vi "MatrixVg_Bdep.vi"(0 "B-table String":string, 3 "Time Stamp":timestamp, 6 "Play Button":bool, 7 "Custom Folder":string, 8 "Settings":T2={"Ring 3"=1, "Ring 2"=4, "Fixed Current mkA"=0.5, "If yes, the current is:"=enum."Radio Selection 1", "Ressitance measurements?"=TRUE, "Commute DC current?"=FALSE} {"Ring 3" items=["1 kOhm", "10 kOhm", "100 kOhm", "1 Mohm", "10 mOhm"]; "Ring 2" items=["1 kOhm", "10 kOhm", "100 kOhm", "1 Mohm", "10 MOhm"]}, 9 "Instruments":T3={"Oscillator"=TRUE, "Addr 1 lock-in"=TRUE, "Addr 1 lock-in oop"=TRUE, "Addr 2 lock-in"=TRUE, "Addr 2 lock-in oop"=TRUE, "Addr 3 lock-in"=FALSE, "Addr 3 lock-in oop"=FALSE, "Voltage (Vk1)"=FALSE, "Current (Ik1)"=TRUE, "Voltage (Vk2)"=FALSE, "Current (Ik2)"=FALSE, "Voltage (Vk3)"=FALSE, "Current (Ik3)"=FALSE, "Channel 1 (Vnano1)  "=FALSE, "Channel 2 (Vnano1b)"=FALSE, "Channel 1 (Vnano2)   "=FALSE, "Channel 2 (Vnano2b)"=FALSE, "Thermometer 1 (T1)"=TRUE, "Magnetic Field (B)"=TRUE, "Capacitance (C) and Loss (L)"=FALSE}, 10 "VgCluster":T4={"V1 (V)"=-1.0, "V2 (V)"=1.0, "Sweep rate, V/min"=1.0, "Time btw \npoints, sec"=1.0, "points at each Vg"=1, "Compliance, mkA"=0.05, "No-record rate, V/min"=30.0, "Full sweep?"=FALSE} {"No-record rate, V/min" min=0.0 max=1.0 step=0.01 format="%_4f"; "V2 (V)" min=-4.0 max=4.0 step=0.1 format="%.1f"; "Compliance, mkA" min=0.0 max=1.0 step=0.01 format="%.3f"; "Time btw \npoints, sec" format="%.2f"; "Sweep rate, V/min" min=0.0 max=1.0 step=0.01 format="%_4f"; "V1 (V)" min=-4.0 max=4.0 step=0.1 format="%.1f"}, 11 "BCluster":T1={"Starting B (T)"=-1.0, "Final B (T)"=1.0, "Step (T)"=1.0, "Time for persistant, min"=1.0} {"Final B (T)" min=-4.0 max=4.0 step=0.1 format="%.2f"; "Time for persistant, min" format="%.2f"; "Step (T)" min=0.0 max=1.0 step=0.01 format="%_4f"; "Starting B (T)" min=-4.0 max=4.0 step=0.1 format="%.2f"}) -> ()   [LabVIEW 2017]
uses:
  <vilib>/Utility/file.llb/Read From Spreadsheet File (DBL).vi
panel:
  out "Communication":string
  out "B Array":dbl[](array[numeric])
  out "Experiment ends at:":string
  out "Hours":dbl format="%.1f"
  out "Estimated time of experiment:":i16
  out "ArraySens":i8[](array[numeric])
  out "ArrayOsc":dbl[](array[numeric])
  out "# of configurations":i8
  out "Large Array":bool[][][](array[boolean])
  out "Contact configuration file (*.conf)":path
  # "hours"
  # "min.="
  # "Values of B field can be also entered as the table by copying\nand pasting a column of numbers in a \"B table\" string at the \nfar right side of this window."
  # "Lock-in Amplifiers"
  # "Temperature"
  # "SourceMeters"
  # "Nanovoltmeters"
  # "Main"
  # "(not recommended, too slow)"
  # "Magnetic Field"
  # "Capacitance & Loss"
  # "(not recommended, too slow)"
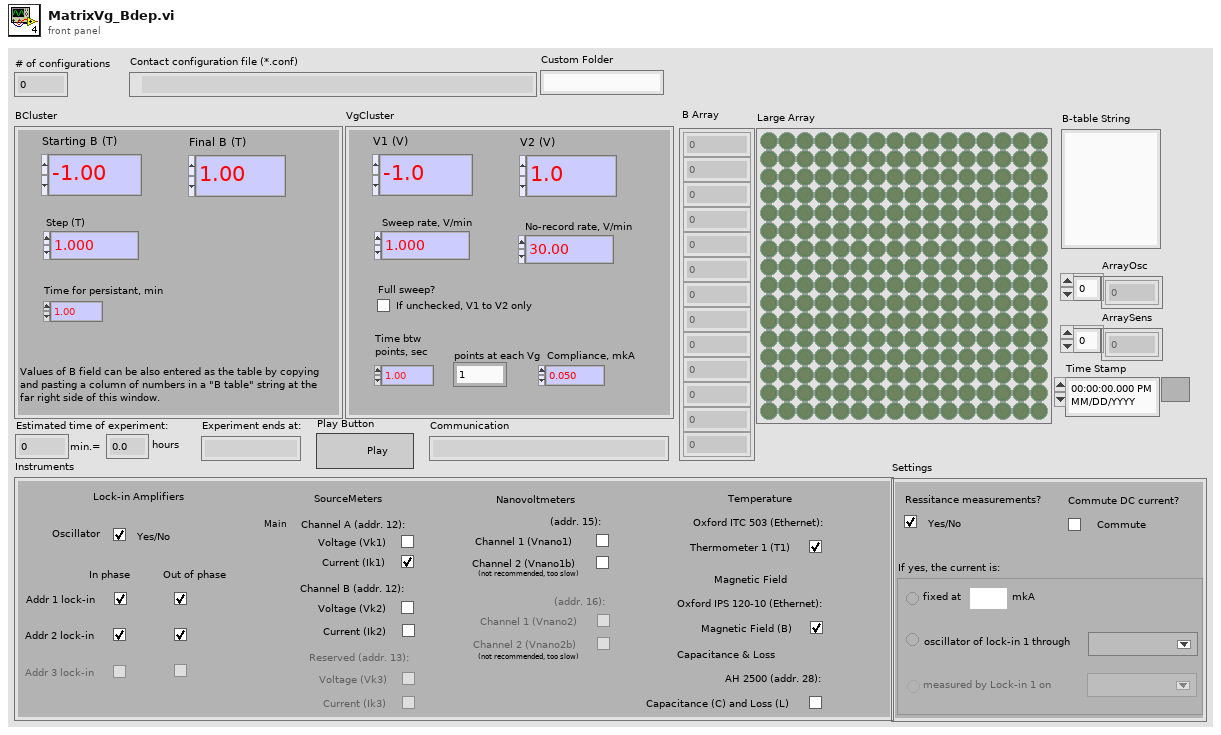
[diagram p1: front panel]
types:
  T1 = cluster{"Starting B (T)":dbl, "Final B (T)":dbl, "Step (T)":dbl, "Time for persistant, min":dbl}
  T2 = cluster{"Ring 3":u16, "Ring 2":u16, "Fixed Current mkA":dbl, "If yes, the current is:":enum32{"Radio Selection 1", "Radio Selection 2", "Radio Selection 3"}, "Ressitance measurements?":bool, "Commute DC current?":bool}
  T3 = cluster{"Oscillator":bool, "Addr 1 lock-in":bool, "Addr 1 lock-in oop":bool, "Addr 2 lock-in":bool, "Addr 2 lock-in oop":bool, "Addr 3 lock-in":bool, "Addr 3 lock-in oop":bool, "Voltage (Vk1)":bool, "Current (Ik1)":bool, "Voltage (Vk2)":bool, "Current (Ik2)":bool, "Voltage (Vk3)":bool, "Current (Ik3)":bool, "Channel 1 (Vnano1)  ":bool, "Channel 2 (Vnano1b)":bool, "Channel 1 (Vnano2)   ":bool, "Channel 2 (Vnano2b)":bool, "Thermometer 1 (T1)":bool, "Magnetic Field (B)":bool, "Capacitance (C) and Loss (L)":bool}
  T4 = cluster{"V1 (V)":dbl, "V2 (V)":dbl, "Sweep rate, V/min":dbl, "Time btw \npoints, sec":dbl, "points at each Vg":i32, "Compliance, mkA":dbl, "No-record rate, V/min":dbl, "Full sweep?":bool}
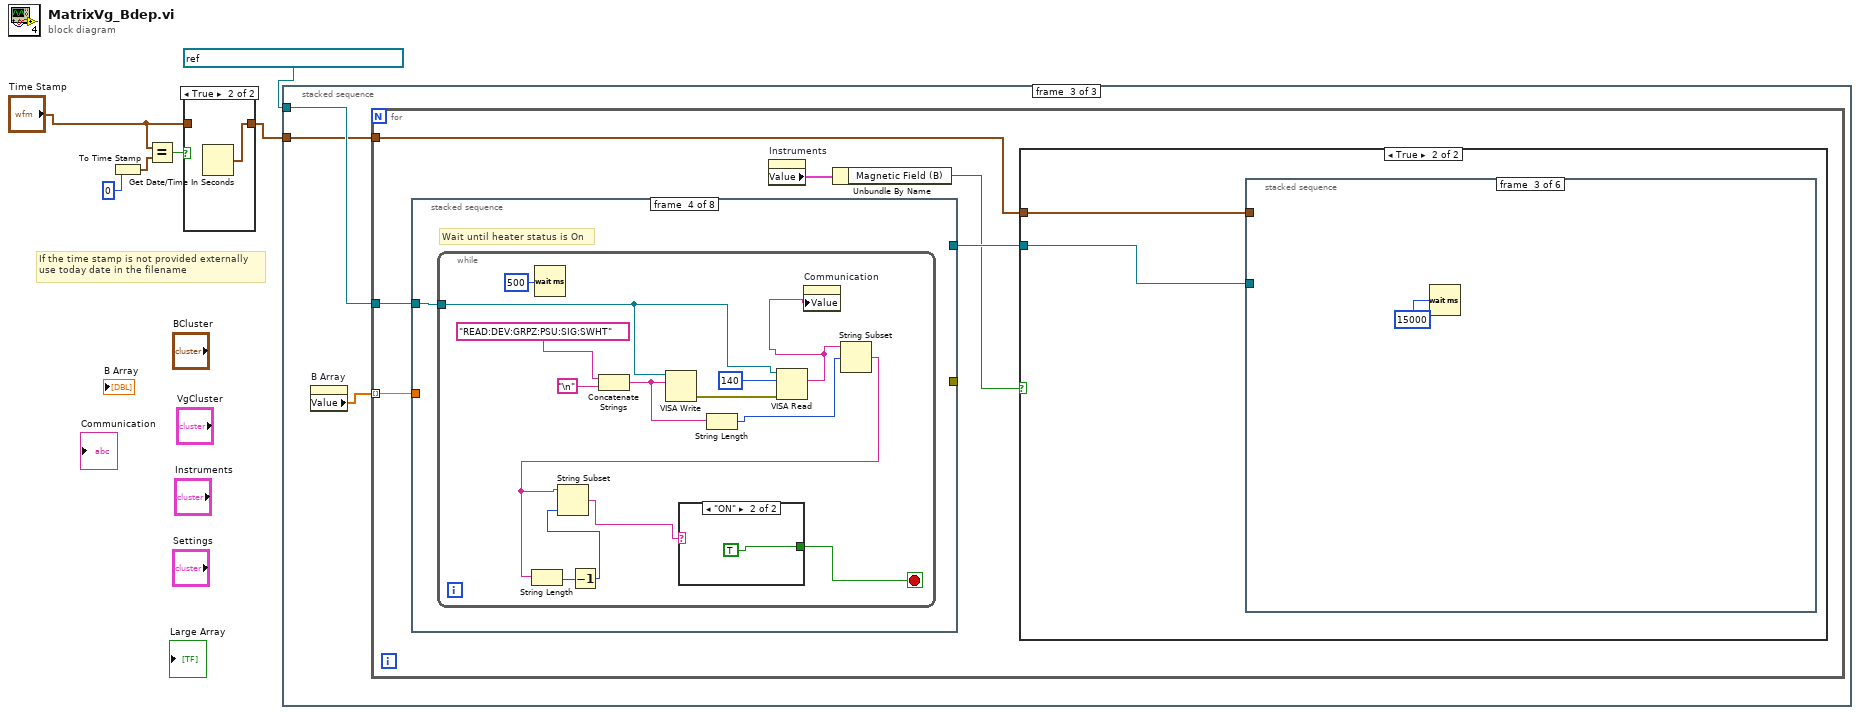
[diagram p0: block diagram]
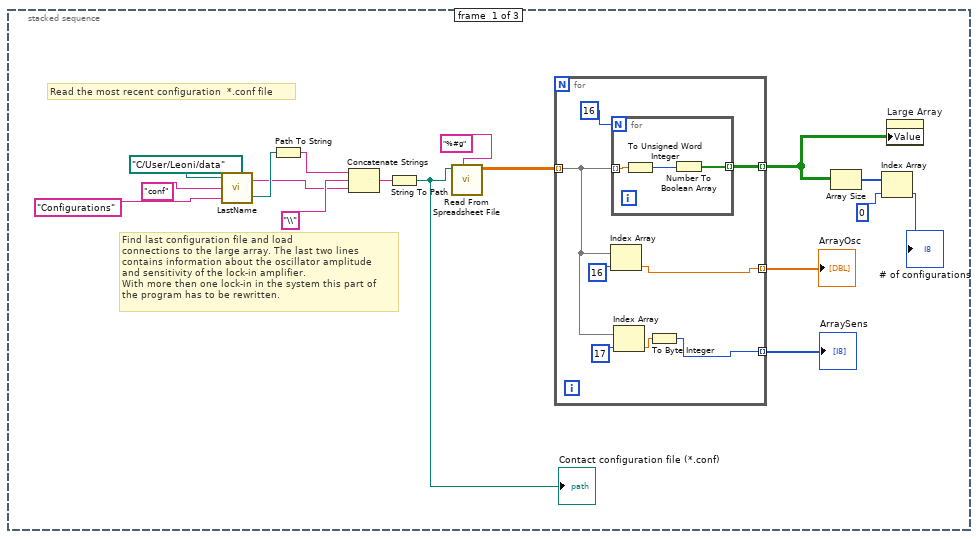
[diagram p3: hidden frame]
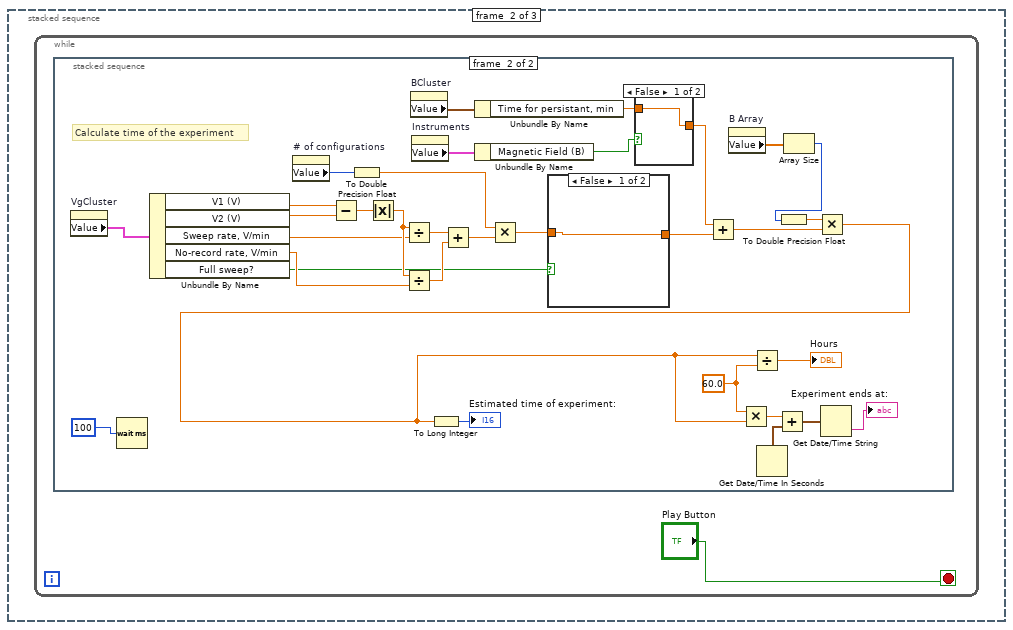
[diagram p4: hidden frame]
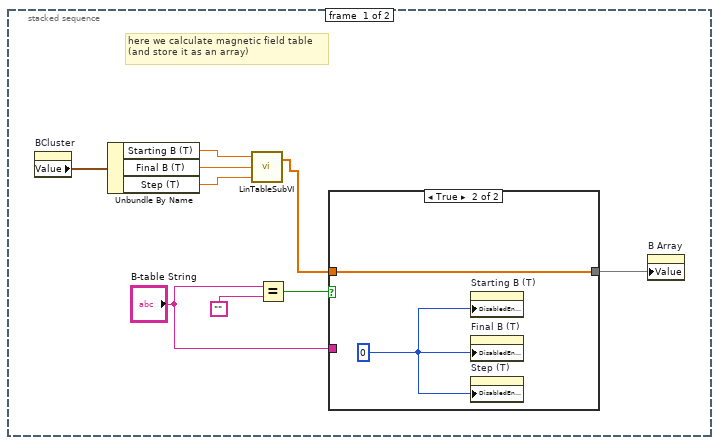
[diagram p5: hidden frame]
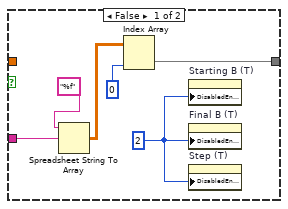
[diagram p6: hidden frame]
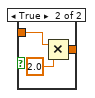
[diagram p7: hidden frame]
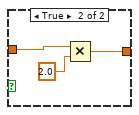
[diagram p8: hidden frame]
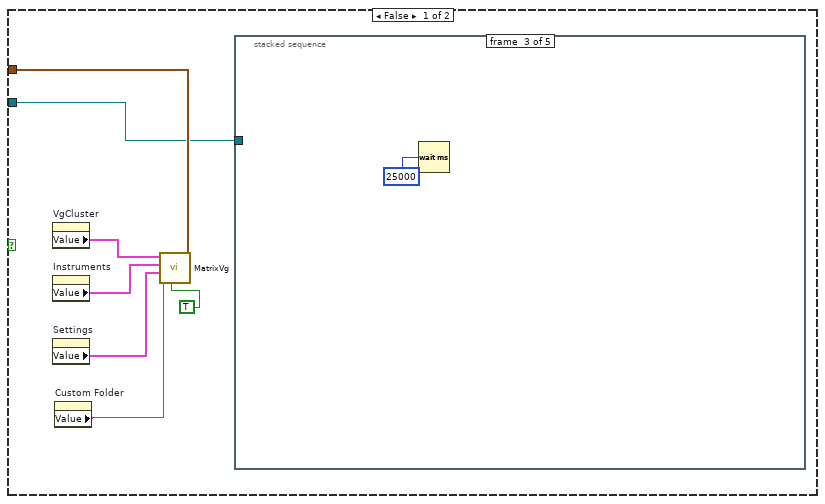
[diagram p9: hidden frame]
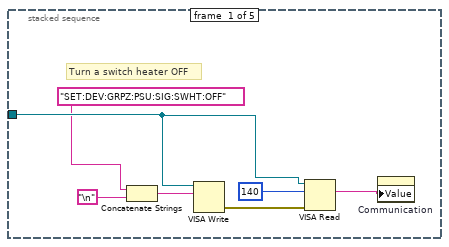
[diagram p10: hidden frame]
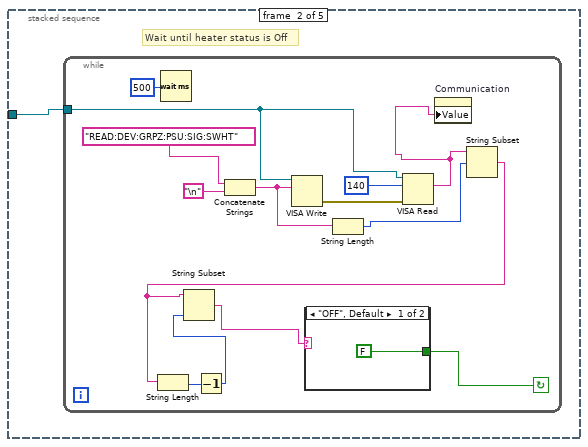
[diagram p11: hidden frame]
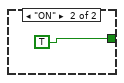
[diagram p12: hidden frame]
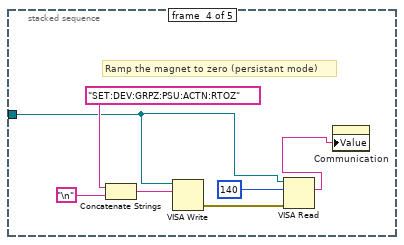
[diagram p13: hidden frame]
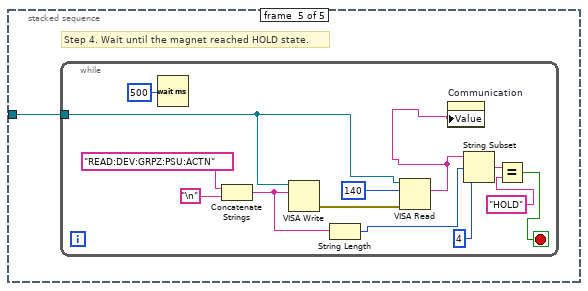
[diagram p14: hidden frame]
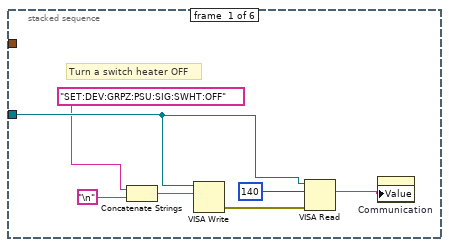
[diagram p15: hidden frame]
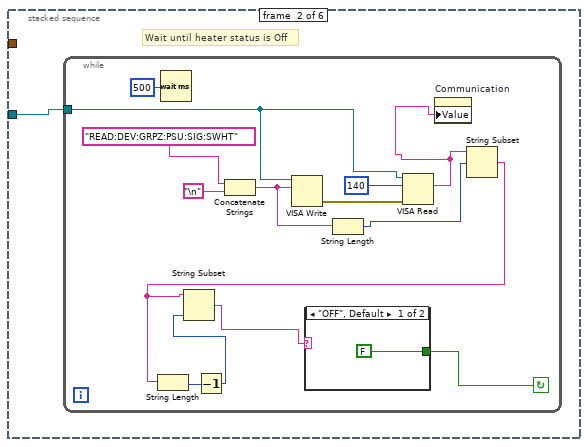
[diagram p16: hidden frame]
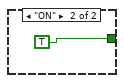
[diagram p17: hidden frame]
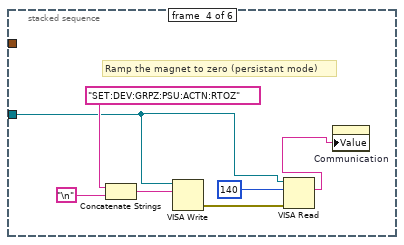
[diagram p18: hidden frame]
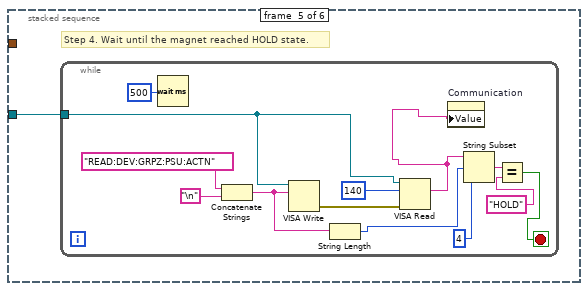
[diagram p19: hidden frame]
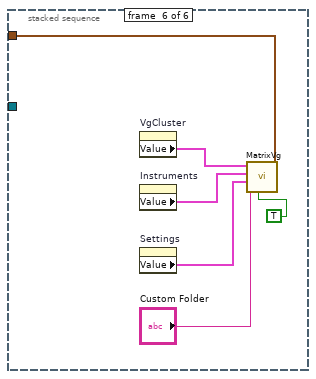
[diagram p20: hidden frame]
diagram:
  # "If the time stamp is not provided externally\nuse today date in the filename"
  n1 = To Time Stamp(1:0) -> (0:w5:timestamp)
  n2 = Equal?(x="Time Stamp", y=w5) -> (x = y?=w4:bool)
  n3 = case shown="True" w4 {
    tunnel: "Time Stamp" -> [w7 _]
    tunnel: [w7 w8] -> w2
    frame False {
    }
    frame True {
      n4 = Get Date/Time In Seconds() -> (seconds since 1Jan1904=w8:timestamp)
    }
  }
  n5 = stacked-sequence {
    tunnel: w2 -> [_ _ w96]
    tunnel: refnum<visa-resource-name> "TCPIP0::192.168.128.3::7020::SOCKET" ("VISA resource name") -> [_ _ w98]
    frame #0 {
      # "Read the most recent configuration  *.conf file"
      # "Find last configuration file and load \nconnections to the large array. The last two lines \ncontains information about the oscillator amplitude\nand sensitivity of the lock-in amplifier.\nWith more then one lock-in in the system this part of \nthe program has to be rewritten."
      n6 = call "LastName.vi"("Custom Folder"="Configurations", "Extention"="conf", "User Data Folder"=path "C:/User/Leoni/data") -> ("created path"=w21:path, "String"=w20:string)
      n7 = Path To String(path=w21) -> (string=w25:string)
      n8 = Concatenate Strings(w25, "\\", w20) -> (w23:string)
      n9 = String To Path(string=w23) -> (path=w11:path)
      "Contact configuration file (*.conf)" <- w11
      n10 = call-poly <vilib>:"Read From Spreadsheet File.vi"("format (%.3f)"="%#g", "file path (dialog if empty)"=w11) -> ("all rows"=w16:dbl[][])  [unwired: 5 in, 4 out]
      n11 = for {
        tunnel: w16 -> [w29] mode=indexing
        tunnel: [w33] -> w13 mode=indexing
        tunnel: [w28] -> w10 mode=indexing
        tunnel: [w27] -> w9 mode=indexing
        n12 = Index Array(array=w29, index=16) -> (element=w28:dbl)
        n13 = for {
          N: 16 -> [_]
          tunnel: w29 -> [w36] mode=indexing
          tunnel: [w34] -> w33 mode=indexing
          n14 = To Unsigned Word Integer(number=w36) -> (unsigned 16bit integer=w35:u16)
          n15 = Number To Boolean Array(number=w35) -> (Boolean array=w34:bool[])
        }
        n16 = Index Array(array=w29, index=17) -> (element=w30:dbl)
        n17 = To Byte Integer(number=w30) -> (8bit integer=w27:i8)
      }
      "ArrayOsc" <- w10
      "ArraySens" <- w9
      n18 = Array Size(array=w13) -> (size(s)=w15:i32[])
      n19 = Index Array(array=w15, index=0) -> (element=→"# of configurations":i32)
      n20 = property on="Large Array" class="Arr (strict)"("Value"=w13) -> ()  [unwired: 2 in, 2 out]
    }
    frame #1 {
      n21 = while {
        stop <- "Play Button" stop-if-true
        n22 = stacked-sequence {
          frame #0 {
            # "here we calculate magnetic field table\n(and store it as an array)"
            n23 = property on="BCluster" class="Clust (strict)"() -> ("Value"=w42:T1)  [unwired: 2 in, 2 out]
            n24 = Unbundle By Name(w42) -> ("Starting B (T)"=w41:dbl, "Final B (T)"=w40:dbl, "Step (T)"=w39:dbl)
            n25 = call "LinTableSubVI.vi"("Step"=w39, "Final"=w40, "Initial"=w41) -> ("Array"=w46:dbl[])  [unwired: 1 in]
            n26 = Equal?(x="B-table String", y="") -> (x = y?=w43:bool)
            n27 = case shown="True" w43 {
              tunnel: [w49 w54] -> w38
              tunnel: w46 -> [_ w54]
              tunnel: "B-table String" -> [w48 _]
              frame False {
                w47 = 2
                n28 = Spreadsheet String To Array(format string="%f", spreadsheet string=w48) -> (array=w51:dbl[][])  [unwired: 2 in]
                n29 = Index Array(array=w51, index (col)=0) -> (element=w49:dbl[])  [unwired: 1 in]
                n30 = property on="Starting B (T)" class="DigNum (strict)"("DisabledEnum"=w47) -> ()  [unwired: 2 in, 2 out]
                n31 = property on="Final B (T)" class="DigNum (strict)"("DisabledEnum"=w47) -> ()  [unwired: 2 in, 2 out]
                n32 = property on="Step (T)" class="DigNum (strict)"("DisabledEnum"=w47) -> ()  [unwired: 2 in, 2 out]
              }
              frame True {
                w53 = 0
                n33 = property on="Starting B (T)" class="DigNum (strict)"("DisabledEnum"=w53) -> ()  [unwired: 2 in, 2 out]
                n34 = property on="Final B (T)" class="DigNum (strict)"("DisabledEnum"=w53) -> ()  [unwired: 2 in, 2 out]
                n35 = property on="Step (T)" class="DigNum (strict)"("DisabledEnum"=w53) -> ()  [unwired: 2 in, 2 out]
              }
            }
            n36 = property on="B Array" class="Arr (strict)"("Value"=w38) -> ()  [unwired: 2 in, 2 out]
          }
          frame #1 {
            w67 = 60.0
            # "Calculate time of the experiment"
            n37 = property on="VgCluster" class="Clust (strict)"() -> ("Value"=w86:T4)  [unwired: 2 in, 2 out]
            n38 = Wait (ms)(milliseconds to wait=100) -> ()  [unwired: 1 out]
            n39 = Unbundle By Name(w86) -> ("V1 (V)"=w85:dbl, "V2 (V)"=w84:dbl, "Sweep rate, V/min"=w81:dbl, "No-record rate, V/min"=w80:dbl, "Full sweep?"=w74:bool)
            n40 = property on="# of configurations" class="DigNum (strict)"() -> ("Value"=w76:i8)  [unwired: 2 in, 2 out]
            n41 = Subtract(x=w85, y=w84) -> (x-y=w83:dbl)
            n42 = To Double Precision Float(number=w76) -> (double precision float=w75:dbl)
            n43 = Absolute Value(x=w83) -> (abs(x)=w82:dbl)
            n44 = Divide(x=w82, y=w81) -> (x/y=w79:dbl)
            n45 = Divide(x=w82, y=w80) -> (x/y=w78:dbl)
            n46 = property on="BCluster" class="Clust (strict)"() -> ("Value"=w63:T1)  [unwired: 2 in, 2 out]
            n47 = property on="Instruments" class="Clust (strict)"() -> ("Value"=w58:T3)  [unwired: 2 in, 2 out]
            n48 = Add(x=w79, y=w78) -> (x+y=w77:dbl)
            n49 = Unbundle By Name(w63) -> ("Time for persistant, min"=w56:dbl)
            n50 = Unbundle By Name(w58) -> ("Magnetic Field (B)"=w57:bool)
            n51 = Multiply(x=w75, y=w77) -> (x*y=w73:dbl)
            n52 = case shown="False" w74 {
              tunnel: w73 -> [w92 w95]
              tunnel: [w92 w93] -> w64
              frame False {
              }
              frame True {
                n53 = Multiply(x=w95, y=2.0) -> (x*y=w93:dbl)
              }
            }
            n54 = case shown="False" w57 {
              tunnel: w56 -> [w88 w90]
              tunnel: [w88 w89] -> w55
              frame False {
              }
              frame True {
                n55 = Multiply(x=w90, y=2.0) -> (x*y=w89:dbl)
              }
            }
            n56 = Add(x=w55, y=w64) -> (x+y=w62:dbl)
            n57 = property on="B Array" class="Arr (strict)"() -> ("Value"=w65:dbl[])  [unwired: 2 in, 2 out]
            n58 = Get Date/Time In Seconds() -> (seconds since 1Jan1904=w71:timestamp)
            n59 = Array Size(array=w65) -> (size(s)=w60:i32)
            n60 = To Double Precision Float(number=w60) -> (double precision float=w61:dbl)
            n61 = Multiply(x=w61, y=w62) -> (x*y=w59:dbl)
            n62 = To Long Integer(number=w59) -> (32bit integer=→"Estimated time of experiment:":i32)
            n63 = Multiply(x=w67, y=w59) -> (x*y=w66:dbl)
            n64 = Divide(x=w59, y=w67) -> (x/y=→"Hours":dbl)
            n65 = Add(x=w66, y=w71) -> (x+y=w70:timestamp)
            n66 = Get Date/Time String(seconds (now)=w70) -> (time string=→"Experiment ends at:":string)  [unwired: 2 in, 1 out]
          }
        }
      }
    }
    frame #2 {
      n67 = property on="B Array" class="Arr (strict)"() -> ("Value"=w97:dbl[])  [unwired: 2 in, 2 out]
      n68 = for {
        tunnel: w98 -> [w104]
        tunnel: w97 -> [w103] mode=indexing
        tunnel: w96 -> [w102]
        n69 = stacked-sequence {
          tunnel: w104 -> [w214 w220 w236 w241 _ w261 w270 w276]
          tunnel: [_ _ _ _ _ _ _ w276] -> w101
          tunnel: w103 -> [_ _ _ _ _ w259 _ _]
          tunnel: [w212 _ _ _ _ _ _ _] -> _
          frame #0 {
            # "Magnet is in a persistant mode.\nRamp the magnet to the set field."
            n70 = Concatenate Strings("SET:DEV:GRPZ:PSU:ACTN:RTOS" ("string"), "\n") -> (w216:string)
            n71 = VISA Write(VISA resource name=w214, write buffer=w216) -> (error out=w219:errorcluster)  [unwired: 1 in, 2 out]
            n72 = VISA Read(VISA resource name=w214, byte count=140, error in (no error)=w219) -> (read buffer=w213:string)  [unwired: 3 out]
            n73 = property on="Communication" class="Str"("Value"=w213) -> (error out=w212:errorcluster)  [unwired: 2 in, 1 out]
          }
          frame #1 {
            # "Wait until the magnet reached HOLD state."
            n74 = while {
              tunnel: w220 -> [w230]
              stop <- w223 stop-if-true
              n75 = Wait (ms)(milliseconds to wait=500) -> ()  [unwired: 1 out]
              n76 = Concatenate Strings("READ:DEV:GRPZ:PSU:ACTN" ("string"), "\n") -> (w227:string)
              n77 = VISA Write(VISA resource name=w230, write buffer=w227) -> (error out=w233:errorcluster)  [unwired: 1 in, 2 out]
              n78 = String Length(string=w227) -> (length=w226:i32)
              n79 = VISA Read(VISA resource name=w230, byte count=140, error in (no error)=w233) -> (read buffer=w221:string)  [unwired: 3 out]
              n80 = property on="Communication" class="Str"("Value"=w221) -> ()  [unwired: 2 in, 2 out]
              n81 = String Subset(string=w221, offset (0)=w226, length (rest)=4) -> (substring=w225:string)
              n82 = Equal?(x=w225, y="HOLD") -> (x = y?=w223:bool)
            }
          }
          frame #2 {
            # "Turn a switch heater ON"
            n83 = Concatenate Strings("SET:DEV:GRPZ:PSU:SIG:SWHT:ON" ("string"), "\n") -> (w237:string)
            n84 = VISA Write(VISA resource name=w236, write buffer=w237) -> (error out=w240:errorcluster)  [unwired: 1 in, 2 out]
            n85 = VISA Read(VISA resource name=w236, byte count=140, error in (no error)=w240) -> (read buffer=w234:string)  [unwired: 3 out]
            n86 = property on="Communication" class="Str"("Value"=w234) -> ()  [unwired: 2 in, 2 out]
          }
          frame #3 {
            # "Wait until heater status is On"
            n87 = while {
              tunnel: w241 -> [w252]
              stop <- w244 stop-if-true
              n88 = Wait (ms)(milliseconds to wait=500) -> ()  [unwired: 1 out]
              n89 = Concatenate Strings("READ:DEV:GRPZ:PSU:SIG:SWHT" ("string"), "\n") -> (w251:string)
              n90 = VISA Write(VISA resource name=w252, write buffer=w251) -> (error out=w255:errorcluster)  [unwired: 1 in, 2 out]
              n91 = String Length(string=w251) -> (length=w250:i32)
              n92 = VISA Read(VISA resource name=w252, byte count=140, error in (no error)=w255) -> (read buffer=w242:string)  [unwired: 3 out]
              n93 = property on="Communication" class="Str"("Value"=w242) -> ()  [unwired: 2 in, 2 out]
              n94 = String Subset(string=w242, offset (0)=w250) -> (substring=w243:string)  [unwired: 1 in]
              n95 = String Length(string=w243) -> (length=w247:i32)
              n96 = Decrement(x=w247) -> (x-1=w246:i32)
              n97 = String Subset(string=w243, length (rest)=w246) -> (substring=w245:string)  [unwired: 1 in]
              n98 = case shown="\"ON\"" w245 {
                tunnel: [FALSE TRUE] -> w244
                frame "OFF", Default {
                }
                frame "ON" {
                }
              }
            }
          }
          frame #4 {
            n99 = Wait (ms)(milliseconds to wait=15000) -> ()  [unwired: 1 out]
          }
          frame #5 {
            # "Set new value of the set field from the tablefield"
            n100 = Number To Fractional String(number=w259) -> (F-format string=w267:string)  [unwired: 3 in]
            n101 = Concatenate Strings("SET:DEV:GRPZ:PSU:SIG:FSET:" ("string"), w267) -> (w262:string)
            n102 = Concatenate Strings(w262, "\n") -> (w263:string)
            n103 = VISA Write(VISA resource name=w261, write buffer=w263) -> (error out=w266:errorcluster)  [unwired: 1 in, 2 out]
            n104 = VISA Read(VISA resource name=w261, byte count=140, error in (no error)=w266) -> (read buffer=w260:string)  [unwired: 3 out]
            n105 = property on="Communication" class="Str"("Value"=w260) -> ()  [unwired: 2 in, 2 out]
          }
          frame #6 {
            # "Ramp the magnet to the new target field"
            n106 = Concatenate Strings("SET:DEV:GRPZ:PSU:ACTN:RTOS" ("string"), "\n") -> (w272:string)
            n107 = VISA Write(VISA resource name=w270, write buffer=w272) -> (error out=w275:errorcluster)  [unwired: 1 in, 2 out]
            n108 = VISA Read(VISA resource name=w270, byte count=140, error in (no error)=w275) -> (read buffer=w269:string)  [unwired: 3 out]
            n109 = property on="Communication" class="Str"("Value"=w269) -> ()  [unwired: 2 in, 2 out]
          }
          frame #7 {
            # "Wait until the magnet reached HOLD state."
            n110 = while {
              tunnel: w276 -> [w286]
              stop <- w279 stop-if-true
              n111 = Wait (ms)(milliseconds to wait=500) -> ()  [unwired: 1 out]
              n112 = Concatenate Strings("READ:DEV:GRPZ:PSU:ACTN" ("string"), "\n") -> (w283:string)
              n113 = VISA Write(VISA resource name=w286, write buffer=w283) -> (error out=w289:errorcluster)  [unwired: 1 in, 2 out]
              n114 = String Length(string=w283) -> (length=w282:i32)
              n115 = VISA Read(VISA resource name=w286, byte count=140, error in (no error)=w289) -> (read buffer=w277:string)  [unwired: 3 out]
              n116 = property on="Communication" class="Str"("Value"=w277) -> ()  [unwired: 2 in, 2 out]
              n117 = String Subset(string=w277, offset (0)=w282, length (rest)=4) -> (substring=w281:string)
              n118 = Equal?(x=w281, y="HOLD") -> (x = y?=w279:bool)
            }
          }
        }
        n119 = property on="Instruments" class="Clust (strict)"() -> ("Value"=w100:T3)  [unwired: 2 in, 2 out]
        n120 = Unbundle By Name(w100) -> ("Magnetic Field (B)"=w99:bool)
        n121 = case shown="True" w99 {
          tunnel: w102 -> [w111 w158]
          tunnel: w101 -> [w110 w159]
          frame False {
            n122 = property on="VgCluster" class="Clust (strict)"() -> ("Value"=w109:T4)  [unwired: 2 in, 2 out]
            n123 = property on="Instruments" class="Clust (strict)"() -> ("Value"=w108:T3)  [unwired: 2 in, 2 out]
            n124 = property on="Settings" class="Clust (strict)"() -> ("Value"=w107:T2)  [unwired: 2 in, 2 out]
            n125 = property on="Custom Folder" class="Str"() -> ("Value"=w105:string)  [unwired: 2 in, 2 out]
            n126 = call "MatrixVg.vi"("Time Stamp"=w111, "Play Button"=TRUE, "Custom Folder"=w105, "Settings"=w107, "Instruments"=w108, "VgCluster"=w109) -> ()  [unwired: 6 in]
            n127 = stacked-sequence {
              tunnel: w110 -> [w114 w119 _ w138 w144]
              frame #0 {
                # "Turn a switch heater OFF"
                n128 = Concatenate Strings("SET:DEV:GRPZ:PSU:SIG:SWHT:OFF" ("string"), "\n") -> (w115:string)
                n129 = VISA Write(VISA resource name=w114, write buffer=w115) -> (error out=w118:errorcluster)  [unwired: 1 in, 2 out]
                n130 = VISA Read(VISA resource name=w114, byte count=140, error in (no error)=w118) -> (read buffer=w112:string)  [unwired: 3 out]
                n131 = property on="Communication" class="Str"("Value"=w112) -> ()  [unwired: 2 in, 2 out]
              }
              frame #1 {
                # "Wait until heater status is Off"
                n132 = while {
                  tunnel: w119 -> [w130]
                  stop <- w122 continue-if-true
                  n133 = Wait (ms)(milliseconds to wait=500) -> ()  [unwired: 1 out]
                  n134 = Concatenate Strings("READ:DEV:GRPZ:PSU:SIG:SWHT" ("string"), "\n") -> (w129:string)
                  n135 = VISA Write(VISA resource name=w130, write buffer=w129) -> (error out=w133:errorcluster)  [unwired: 1 in, 2 out]
                  n136 = String Length(string=w129) -> (length=w128:i32)
                  n137 = VISA Read(VISA resource name=w130, byte count=140, error in (no error)=w133) -> (read buffer=w120:string)  [unwired: 3 out]
                  n138 = property on="Communication" class="Str"("Value"=w120) -> ()  [unwired: 2 in, 2 out]
                  n139 = String Subset(string=w120, offset (0)=w128) -> (substring=w121:string)  [unwired: 1 in]
                  n140 = String Length(string=w121) -> (length=w125:i32)
                  n141 = Decrement(x=w125) -> (x-1=w124:i32)
                  n142 = String Subset(string=w121, length (rest)=w124) -> (substring=w123:string)  [unwired: 1 in]
                  n143 = case shown="\"OFF\", Default" w123 {
                    tunnel: [FALSE TRUE] -> w122
                    frame "OFF", Default {
                    }
                    frame "ON" {
                    }
                  }
                }
              }
              frame #2 {
                n144 = Wait (ms)(milliseconds to wait=25000) -> ()  [unwired: 1 out]
              }
              frame #3 {
                # "Ramp the magnet to zero (persistant mode)"
                n145 = Concatenate Strings("SET:DEV:GRPZ:PSU:ACTN:RTOZ" ("string"), "\n") -> (w140:string)
                n146 = VISA Write(VISA resource name=w138, write buffer=w140) -> (error out=w143:errorcluster)  [unwired: 1 in, 2 out]
                n147 = VISA Read(VISA resource name=w138, byte count=140, error in (no error)=w143) -> (read buffer=w137:string)  [unwired: 3 out]
                n148 = property on="Communication" class="Str"("Value"=w137) -> ()  [unwired: 2 in, 2 out]
              }
              frame #4 {
                # "Step 4. Wait until the magnet reached HOLD state."
                n149 = while {
                  tunnel: w144 -> [w154]
                  stop <- w145 stop-if-true
                  n150 = Wait (ms)(milliseconds to wait=500) -> ()  [unwired: 1 out]
                  n151 = Concatenate Strings("READ:DEV:GRPZ:PSU:ACTN" ("string"), "\n") -> (w151:string)
                  n152 = VISA Write(VISA resource name=w154, write buffer=w151) -> (error out=w157:errorcluster)  [unwired: 1 in, 2 out]
                  n153 = String Length(string=w151) -> (length=w150:i32)
                  n154 = VISA Read(VISA resource name=w154, byte count=140, error in (no error)=w157) -> (read buffer=w146:string)  [unwired: 3 out]
                  n155 = property on="Communication" class="Str"("Value"=w146) -> ()  [unwired: 2 in, 2 out]
                  n156 = String Subset(string=w146, offset (0)=w150, length (rest)=4) -> (substring=w149:string)
                  n157 = Equal?(x=w149, y="HOLD") -> (x = y?=w145:bool)
                }
              }
            }
          }
          frame True {
            n158 = stacked-sequence {
              tunnel: w159 -> [w162 w167 _ w186 w192 _]
              tunnel: w158 -> [_ _ _ _ _ w206]
              frame #0 {
                # "Turn a switch heater OFF"
                n159 = Concatenate Strings("SET:DEV:GRPZ:PSU:SIG:SWHT:OFF" ("string"), "\n") -> (w163:string)
                n160 = VISA Write(VISA resource name=w162, write buffer=w163) -> (error out=w166:errorcluster)  [unwired: 1 in, 2 out]
                n161 = VISA Read(VISA resource name=w162, byte count=140, error in (no error)=w166) -> (read buffer=w160:string)  [unwired: 3 out]
                n162 = property on="Communication" class="Str"("Value"=w160) -> ()  [unwired: 2 in, 2 out]
              }
              frame #1 {
                # "Wait until heater status is Off"
                n163 = while {
                  tunnel: w167 -> [w178]
                  stop <- w170 continue-if-true
                  n164 = Wait (ms)(milliseconds to wait=500) -> ()  [unwired: 1 out]
                  n165 = Concatenate Strings("READ:DEV:GRPZ:PSU:SIG:SWHT" ("string"), "\n") -> (w177:string)
                  n166 = VISA Write(VISA resource name=w178, write buffer=w177) -> (error out=w181:errorcluster)  [unwired: 1 in, 2 out]
                  n167 = String Length(string=w177) -> (length=w176:i32)
                  n168 = VISA Read(VISA resource name=w178, byte count=140, error in (no error)=w181) -> (read buffer=w168:string)  [unwired: 3 out]
                  n169 = property on="Communication" class="Str"("Value"=w168) -> ()  [unwired: 2 in, 2 out]
                  n170 = String Subset(string=w168, offset (0)=w176) -> (substring=w169:string)  [unwired: 1 in]
                  n171 = String Length(string=w169) -> (length=w173:i32)
                  n172 = Decrement(x=w173) -> (x-1=w172:i32)
                  n173 = String Subset(string=w169, length (rest)=w172) -> (substring=w171:string)  [unwired: 1 in]
                  n174 = case shown="\"OFF\", Default" w171 {
                    tunnel: [FALSE TRUE] -> w170
                    frame "OFF", Default {
                    }
                    frame "ON" {
                    }
                  }
                }
              }
              frame #2 {
                n175 = Wait (ms)(milliseconds to wait=15000) -> ()  [unwired: 1 out]
              }
              frame #3 {
                # "Ramp the magnet to zero (persistant mode)"
                n176 = Concatenate Strings("SET:DEV:GRPZ:PSU:ACTN:RTOZ" ("string"), "\n") -> (w188:string)
                n177 = VISA Write(VISA resource name=w186, write buffer=w188) -> (error out=w191:errorcluster)  [unwired: 1 in, 2 out]
                n178 = VISA Read(VISA resource name=w186, byte count=140, error in (no error)=w191) -> (read buffer=w185:string)  [unwired: 3 out]
                n179 = property on="Communication" class="Str"("Value"=w185) -> ()  [unwired: 2 in, 2 out]
              }
              frame #4 {
                # "Step 4. Wait until the magnet reached HOLD state."
                n180 = while {
                  tunnel: w192 -> [w202]
                  stop <- w193 stop-if-true
                  n181 = Wait (ms)(milliseconds to wait=500) -> ()  [unwired: 1 out]
                  n182 = Concatenate Strings("READ:DEV:GRPZ:PSU:ACTN" ("string"), "\n") -> (w199:string)
                  n183 = VISA Write(VISA resource name=w202, write buffer=w199) -> (error out=w205:errorcluster)  [unwired: 1 in, 2 out]
                  n184 = String Length(string=w199) -> (length=w198:i32)
                  n185 = VISA Read(VISA resource name=w202, byte count=140, error in (no error)=w205) -> (read buffer=w194:string)  [unwired: 3 out]
                  n186 = property on="Communication" class="Str"("Value"=w194) -> ()  [unwired: 2 in, 2 out]
                  n187 = String Subset(string=w194, offset (0)=w198, length (rest)=4) -> (substring=w197:string)
                  n188 = Equal?(x=w197, y="HOLD") -> (x = y?=w193:bool)
                }
              }
              frame #5 {
                n189 = property on="VgCluster" class="Clust (strict)"() -> ("Value"=w211:T4)  [unwired: 2 in, 2 out]
                n190 = property on="Instruments" class="Clust (strict)"() -> ("Value"=w210:T3)  [unwired: 2 in, 2 out]
                n191 = property on="Settings" class="Clust (strict)"() -> ("Value"=w209:T2)  [unwired: 2 in, 2 out]
                n192 = call "MatrixVg.vi"("Time Stamp"=w206, "Play Button"=TRUE, "Custom Folder"="Custom Folder", "Settings"=w209, "Instruments"=w210, "VgCluster"=w211) -> ()  [unwired: 6 in]
              }
            }
          }
        }
      }
    }
  }
